vi "23384_Davis_Poku_Amankwa_Amankwa.DavisPoku.MNE1201.8.8_348265_201780221.vi"() -> ()   [LabVIEW 2018]
panel:
  out "Time to press OK[s]":dbl
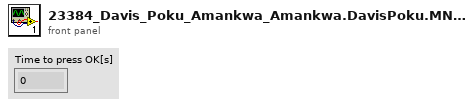
[diagram p1: front panel]
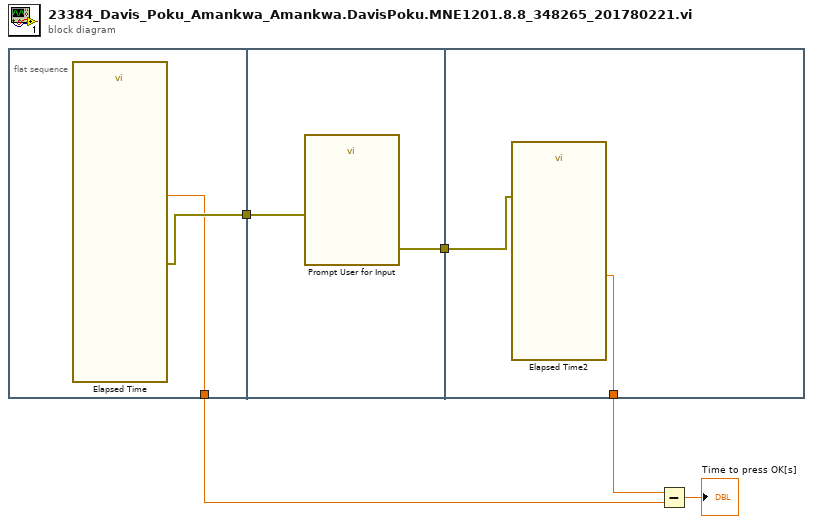
[diagram p0: block diagram]
diagram:
  n1 = flat-sequence {
    tunnel: [w7] -> w5
    tunnel: [w6] -> w3
    tunnel: w5 -> [w9]
    tunnel: [w8] -> w4
    tunnel: w4 -> [w11]
    tunnel: [w10] -> w2
    frame #0 {
      n2 = call "Elapsed Time"() -> ("Present (s)"=w6:dbl, "error out"=w7:errorcluster)  [unwired: 12 in, 6 out]
    }
    frame #1 {
      n3 = call "Prompt User for Input"("error in (no error)"=w9) -> ("error out"=w8:errorcluster)  [unwired: 17 in, 1 out]
    }
    frame #2 {
      n4 = call "Elapsed Time2"("error in (no error)"=w11) -> ("Present (s)"=w10:dbl)  [unwired: 11 in, 7 out]
    }
  }
  n5 = Subtract(x=w2, y=w3) -> (x-y=→"Time to press OK[s]":dbl)
